vi "Set Editor.vi"(8 "error in":errorcluster, 10 "Editor Control Base":refnum<class "Editor Control Base.lvclass">, 11 "Cell in":refnum<class "Cell.lvclass">) -> (0 "error out":errorcluster, 3 "Cell out":refnum<class "Cell.lvclass">)   [LabVIEW 2024, in "SourceGrid.lvlib" / "Cell.lvclass"]
uses:
  Cell.lvclass
  Editors/Editor Base/Editor Control Base.lvclass
  Cell.lvclass/Cell.ctl
  D:/git/Sourcegrid-LabVIEW/dll/SourceGrid.dll
  dll/SourceGrid.dll
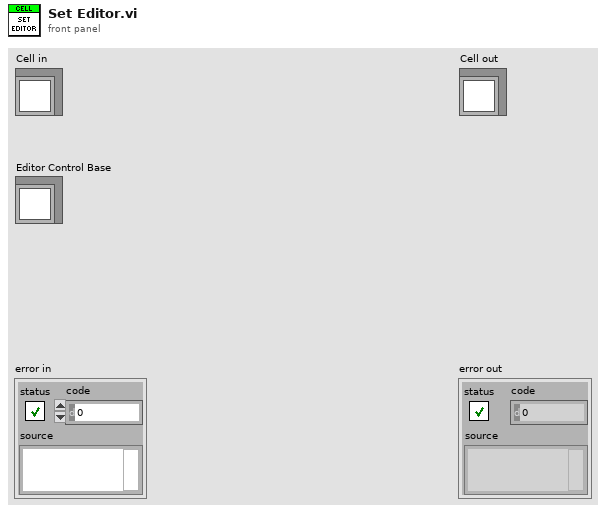
[diagram p1: front panel]
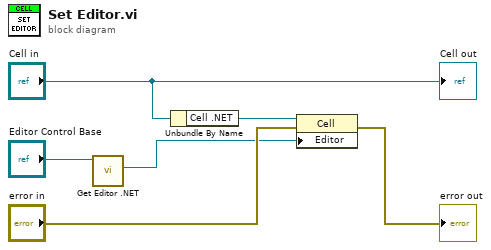
[diagram p0: block diagram]
diagram:
  n1 = call-dynamic "Get Editor .NET.vi"("Editor Control Base in"="Editor Control Base") -> ("Editor Control .NET"=w1:refnum<k24>)  [unwired: 9 in, 1 out]
  n2 = Unbundle By Name("Cell in") -> ("Cell .NET"=w5:refnum<k24>)
  n3 = property class="Cell"(reference=w5, error in="error in", "Editor"=w1) -> (error out=→"error out":errorcluster)  [unwired: 1 out]
  "Cell out" <- "Cell in"
